vi "MagHistString to Shot Data.vi"(8 "error in (no error)":errorcluster, 11 "String":string) -> (0 "error out":errorcluster, 3 "Shot data":T1)   [LabVIEW 2015]
uses:
  Shot data.ctl
  <vilib>/Utility/miscctls.llb/LVDateTimeRec.ctl
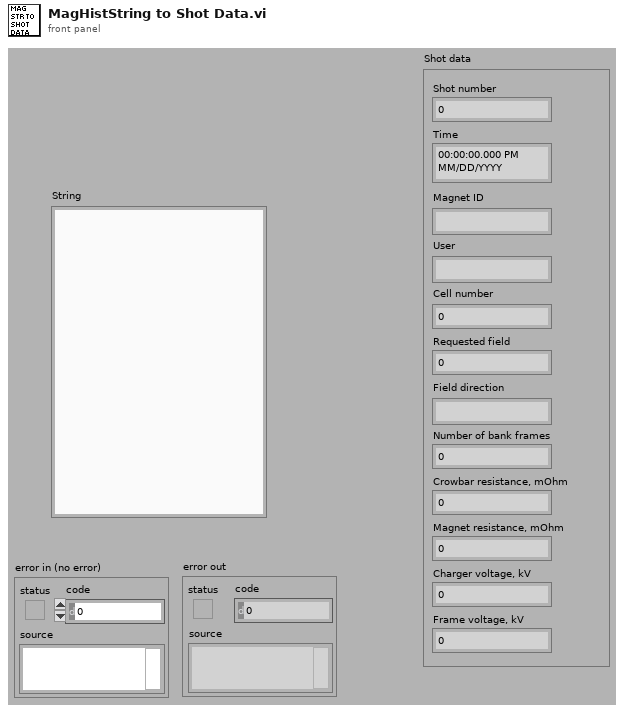
[diagram p1: front panel]
types:
  T1 = typedef "Shot data.ctl" = cluster{"Shot number":i32, "Time":timestamp, "Magnet ID":string, "User":string, "Cell number":i32, "Requested field":dbl, "Field direction":string, "Number of bank frames":i32, "Crowbar resistance, mOhm":dbl, "Magnet resistance, mOhm":dbl, "Charger voltage, kV":dbl, "Frame voltage, kV":dbl}
  T2 = typedef "LVDateTimeRec.ctl" = cluster{"fractional second":dbl, "second":i32, "minute":i32, "hour":i32, "day of month":i32, "month":i32, "year":i32, "day of week":i32, "day of year":i32, "DST":i32}
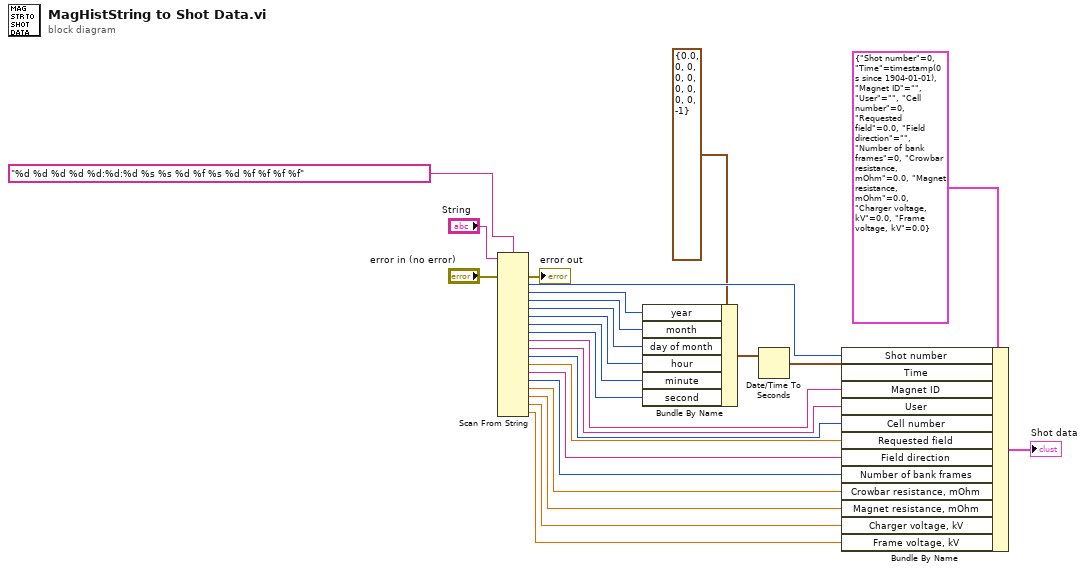
[diagram p0: block diagram]
diagram:
  n1 = Scan From String(format string="%d %d %d %d %d:%d:%d %s %s %d %f %s %d %f %f %f %f", input string="String", error in="error in (no error)") -> (error out=→"error out":errorcluster, output 1=w22:i32, output 2=w8:i32, output 3=w7:i32, output 4=w6:i32, output 5=w4:i32, output 6=w3:i32, output 7=w2:i32, output 8=w20:string, output 9=w19:string, output 10=w18:i32, output 11=w17:dbl, output 12=w16:string, output 13=w15:i32, output 14=w14:dbl, output 15=w13:dbl, output 16=w12:dbl, output 17=w11:dbl)  [unwired: 18 in, 2 out]
  n2 = Bundle By Name(cluster=T2 {"fractional second"=0.0, "second"=0, "minute"=0, "hour"=0, "day of month"=0, "month"=0, "year"=0, "day of week"=0, "day of year"=0, "DST"=-1} ("date time rec"), "year"=w8, "month"=w7, "day of month"=w6, "hour"=w4, "minute"=w3, "second"=w2) -> (w9:T2)
  n3 = Date/Time To Seconds(2:w9) -> (0:w5:timestamp)  [unwired: 1 in]
  n4 = Bundle By Name(cluster=T1 {"Shot number"=0, "Time"=timestamp(0 s since 1904-01-01), "Magnet ID"="", "User"="", "Cell number"=0, "Requested field"=0.0, "Field direction"="", "Number of bank frames"=0, "Crowbar resistance, mOhm"=0.0, "Magnet resistance, mOhm"=0.0, "Charger voltage, kV"=0.0, "Frame voltage, kV"=0.0} ("Shot data"), "Shot number"=w22, "Time"=w5, "Magnet ID"=w20, "User"=w19, "Cell number"=w18, "Requested field"=w17, "Field direction"=w16, "Number of bank frames"=w15, "Crowbar resistance, mOhm"=w14, "Magnet resistance, mOhm"=w13, "Charger voltage, kV"=w12, "Frame voltage, kV"=w11) -> (→"Shot data":T1)
